vi "In Shooting Position.vi"() -> (0 "In Shoot Position":bool)   [LabVIEW 2011]
uses:
  Robot Global Data.vi
panel:
  in  "Desired X Range":cluster{dbl, dbl}(slide) scale=-1.0..1.0
  in  "Desired Y Range":cluster{dbl, dbl}(slide) scale=-1.0..1.0
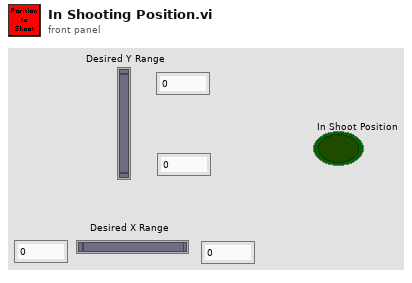
[diagram p1: front panel]
types:
  T1 = cluster{"Position":cluster{"X":dbl, "Y":dbl}, "Distance (ft)":dbl, "Angle Offset":dbl, "Bounding Box":cluster{"Left":dbl, "Top":dbl, "Right":dbl, "Bottom":dbl}}[]
  T2 = cluster{"Position":cluster{"X":dbl, "Y":dbl}, "Distance (ft)":dbl, "Angle Offset":dbl, "Bounding Box":cluster{"Left":dbl, "Top":dbl, "Right":dbl, "Bottom":dbl}}
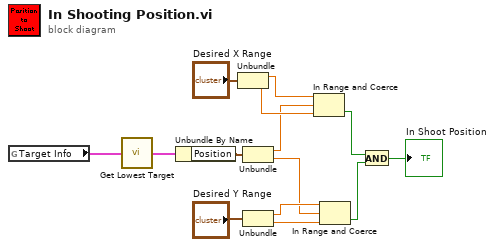
[diagram p0: block diagram]
diagram:
  n1 = global read "Robot Global Data.vi" "Target Info"() -> (w14:T1)
  n2 = call "Get Lowest Target.vi"("Target Info"=w14) -> ("Lowest Target Info"=w13:T2)
  n3 = Unbundle By Name(w13) -> ("Position"=w12:cluster{"X":dbl, "Y":dbl})
  n4 = Unbundle("Desired X Range") -> (w9:dbl, w8:dbl)
  n5 = Unbundle(w12) -> ("X"=w7:dbl, "Y"=w4:dbl)
  n6 = Unbundle("Desired Y Range") -> (w6:dbl, w5:dbl)
  n7 = In Range and Coerce(upper limit=w9, x=w7, lower limit=w8) -> (In Range?=w3:bool)  [unwired: 1 out]
  n8 = In Range and Coerce(upper limit=w6, x=w4, lower limit=w5) -> (In Range?=w2:bool)  [unwired: 1 out]
  n9 = And(x=w3, y=w2) -> (x .and. y?=→"In Shoot Position":bool)
